vi "novatel_bestvel.vi"(11 "gps_data":u8[](array[numeric])=[170, 68, 18, 28, 42, 0, 2, 32, 72, 0, 0, 0, 144, 180, 147, 5, 176, 171, 185, 18, 0, 0, 0, 0, 69, 97, 188, 10, 0, 0, 0, 0, 16, 0, 0, 0, 27, 4, 80, 179, 242, 142, 73, 64, 22, 250, 107, 190, 124, 130, 92, 192, 0, 96, 118, 159, 68, 159, 144, 64, 166, 42, 130, 193, 61, 0, 0, 0, 18, 90, 203, 63, 205, 158, 152, 63, 219, 102, 64, 64, 0, 48, 48, 48, 0, 0, 0, 0, 0, 0, 0, 0, 11, 11, 0, 0, 0, 6, 0, 3, 66, 220, 76, 72]) -> (3 "vel":dbl[](array[numeric]) format="%#_19f")   [LabVIEW 2015]
panel:
  out "checksum":bool
  out "bestvel":T1 {"sol stat" format="%x"; "vel type" format="%x"}
  out "log Header":T2 {"Sync_AA" format="%02x"; "Sync_44" format="%02x"; "Sync_12" format="%02x"; "Message ID" format="%.6f"; "ms" format="%.19f"}
  out "error out":errorcluster
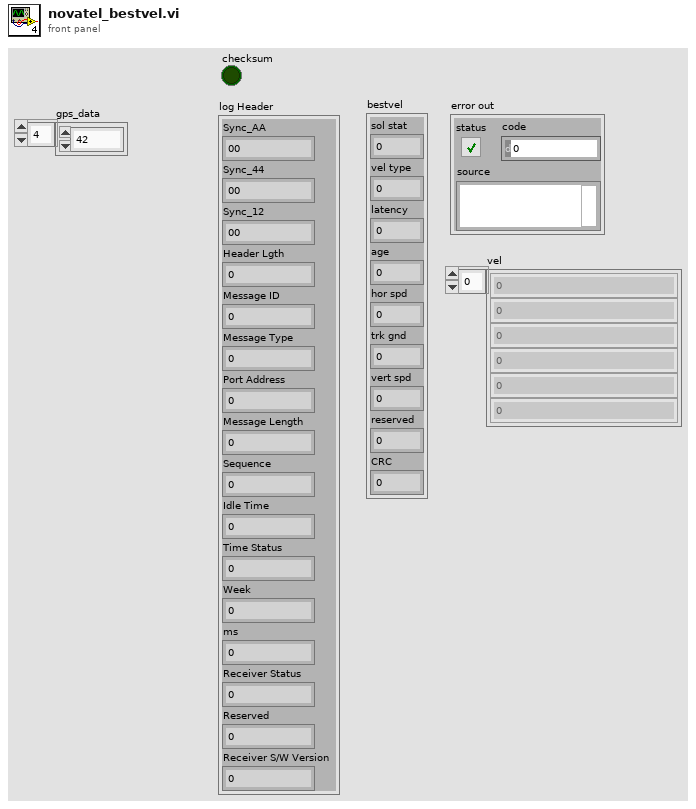
[diagram p1: front panel]
types:
  T1 = cluster{"sol stat":u32, "vel type":u32, "latency":sgl, "age":sgl, "hor spd":dbl, "trk gnd":dbl, "vert spd":dbl, "reserved":sgl, "CRC":u32}
  T2 = cluster{"Sync_AA":u8, "Sync_44":u8, "Sync_12":u8, "Header Lgth":u8, "Message ID":u16, "Message Type":u8, "Port Address":u8, "Message Length":u16, "Sequence":u16, "Idle Time":u8, "Time Status":u8, "Week":u16, "ms":u32, "Receiver Status":u32, "Reserved":u16, "Receiver S/W Version":u16}
  T3 = enum16{"big-endian, network order", "native, host order", "little-endian"}
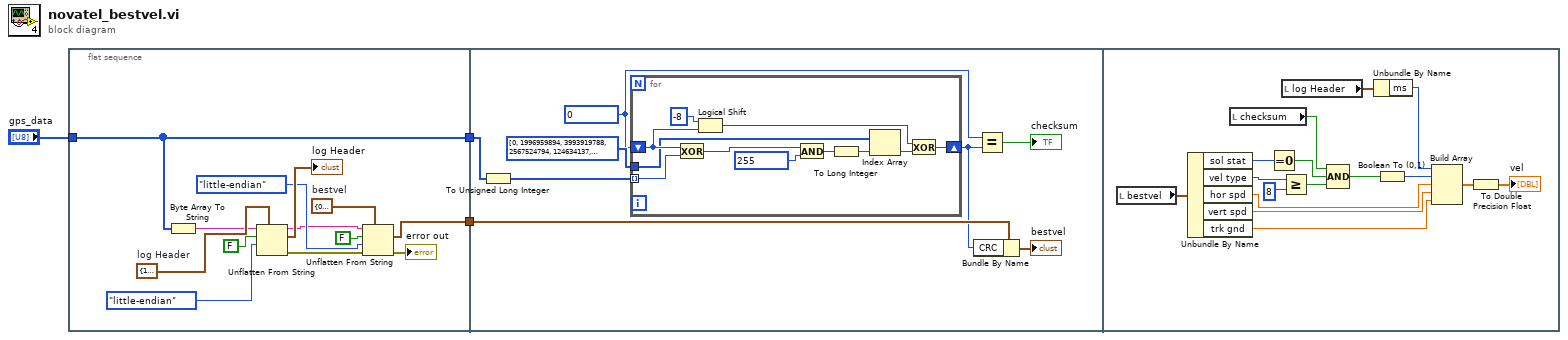
[diagram p0: block diagram]
diagram:
  n1 = flat-sequence {
    tunnel: "gps_data" -> [w7]
    tunnel: [w7] -> w3
    tunnel: [w6] -> w2
    tunnel: w3 -> [w18]
    tunnel: w2 -> [w20]
    frame #0 {
      w4 = T1 {"sol stat"=0, "vel type"=0, "latency"=0.0, "age"=0.0, "hor spd"=0.0, "trk gnd"=0.0, "vert spd"=0.0, "reserved"=0.0, "CRC"=0}  # bestvel
      w16 = T2 {"Sync_AA"=170, "Sync_44"=68, "Sync_12"=18, "Header Lgth"=0, "Message ID"=0, "Message Type"=0, "Port Address"=0, "Message Length"=0, "Sequence"=0, "Idle Time"=0, "Time Status"=0, "Week"=0, "ms"=0, "Receiver Status"=0, "Reserved"=0, "Receiver S/W Version"=0}  # log Header
      n2 = Byte Array To String(unsigned byte array=w7) -> (string=w13:string)
      n3 = Unflatten From String(type=w16, binary string=w13, data includes array or string size? (T)=FALSE, byte order (0:big-endian, network order)=T3."little-endian") -> (rest of the binary string=w10:string, value=→"log Header":T2, error out=w8:errorcluster)  [unwired: 1 in]
      n4 = Unflatten From String(type=w4, binary string=w10, data includes array or string size? (T)=FALSE, byte order (0:big-endian, network order)=T3."little-endian", error in (no error)=w8) -> (value=w6:T1, error out=→"error out":errorcluster)  [unwired: 1 out]
    }
    frame #1 {
      w22 = u32 0
      n5 = To Unsigned Long Integer(number=w18) -> (unsigned 32bit integer=w24:u32[])
      n6 = for {
        shift-right: [w31] -> w19
        shift-left: w22 -> [w34]
        tunnel: w24 -> [w29] mode=indexing
        tunnel: u32[] [0, 1996959894, 3993919788, 2567524794, 124634137, 1886057615, 3915621685, 2657392035, 249268274, 2044508324, 3772115230, 2547177864, 162941995, 2125561021, 3887607047, 2428444049, 498536548, 1789927666, 4089016648, 2227061214, 450548861, 1843258603, 4107580753, 2211677639, 325883990, 1684777152, 4251122042, 2321926636, 335633487, 1661365465, 4195302755, 2366115317, 997073096, 1281953886, 3579855332, 2724688242, 1006888145, 1258607687, 3524101629, 2768942443, 901097722, 1119000684, 3686517206, 2898065728, 853044451, 1172266101, 3705015759, 2882616665, 651767980, 1373503546, 3369554304, 3218104598, 565507253, 1454621731, 3485111705, 3099436303, 671266974, 1594198024, 3322730930, 2970347812, 795835527, 1483230225, 3244367275, 3060149565, 1994146192, 31158534, 2563907772, 4023717930, 1907459465, 112637215, 2680153253, 3904427059, 2013776290, 251722036, 2517215374, 3775830040, 2137656763, 141376813, 2439277719, 3865271297, 1802195444, 476864866, 2238001368, 4066508878, 1812370925, 453092731, 2181625025, 4111451223, 1706088902, 314042704, 2344532202, 4240017532, 1658658271, 366619977, 2362670323, 4224994405, 1303535960, 984961486, 2747007092, 3569037538, 1256170817, 1037604311, 2765210733, 3554079995, 1131014506, 879679996, 2909243462, 3663771856, 1141124467, 855842277, 2852801631, 3708648649, 1342533948, 654459306, 3188396048, 3373015174, 1466479909, 544179635, 3110523913, 3462522015, 1591671054, 702138776, 2966460450, 3352799412, 1504918807, 783551873, 3082640443, 3233442989, 3988292384, 2596254646, 62317068, 1957810842, 3939845945, 2647816111, 81470997, 1943803523, 3814918930, 2489596804, 225274430, 2053790376, 3826175755, 2466906013, 167816743, 2097651377, 4027552580, 2265490386, 503444072, 1762050814, 4150417245, 2154129355, 426522225, 1852507879, 4275313526, 2312317920, 282753626, 1742555852, 4189708143, 2394877945, 397917763, 1622183637, 3604390888, 2714866558, 953729732, 1340076626, 3518719985, 2797360999, 1068828381, 1219638859, 3624741850, 2936675148, 906185462, 1090812512, 3747672003, 2825379669, 829329135, 1181335161, 3412177804, 3160834842, 628085408, 1382605366, 3423369109, 3138078467, 570562233, 1426400815, 3317316542, 2998733608, 733239954, 1555261956, 3268935591, 3050360625, 752459403, 1541320221, 2607071920, 3965973030, 1969922972, 40735498, 2617837225, 3943577151, 1913087877, 83908371, 2512341634, 3803740692, 2075208622, 213261112, 2463272603, 3855990285, 2094854071, 198958881, 2262029012, 4057260610, 1759359992, 534414190, 2176718541, 4139329115, 1873836001, 414664567, 2282248934, 4279200368, 1711684554, 285281116, 2405801727, 4167216745, 1634467795, 376229701, 2685067896, 3608007406, 1308918612, 956543938, 2808555105, 3495958263, 1231636301, 1047427035, 2932959818, 3654703836, 1088359270, 936918000, 2847714899, 3736837829, 1202900863, 817233897, 3183342108, 3401237130, 1404277552, 615818150, 3134207493, 3453421203, 1423857449, 601450431, 3009837614, 3294710456, 1567103746, 711928724, 3020668471, 3272380065, 1510334235, 755167117] ("Array") -> [w25]
        n7 = Exclusive Or(1:w29, 2:w34) -> (0:w33:u32)
        n8 = Logical Shift(y=i16 -8, x=w34) -> (x << y=w30:u32)
        n9 = And(x=w33, y=u32 255) -> (x .and. y?=w28:u32)
        n10 = To Long Integer(number=w28) -> (32bit integer=w27:i32)
        n11 = Index Array(array=w25, index=w27) -> (element=w26:u32)
        n12 = Exclusive Or(1:w26, 2:w30) -> (0:w31:u32)
      }
      n13 = Bundle By Name(cluster=w20, "CRC"=w19) -> (→"bestvel":T1)
      n14 = Equal?(x=w22, y=w19) -> (x = y?=→"checksum":bool)
    }
    frame #2 {
      n15 = local read "bestvel"() -> (w43:T1)
      n16 = Unbundle By Name(w43) -> ("sol stat"=w42:u32, "vel type"=w41:u32, "hor spd"=w51:dbl, "vert spd"=w50:dbl, "trk gnd"=w49:dbl)
      n17 = local read "checksum"() -> (w40:bool)
      n18 = Equal To 0?(x=w42) -> (x = 0?=w39:bool)
      n19 = Greater Or Equal?(x=w41, y=u32 8) -> (x >= y?=w38:bool)
      n20 = local read "log Header"() -> (w47:T2)
      n21 = Compound Arithmetic op=AND(w40, w39, w38) -> (w37:bool)
      n22 = Unbundle By Name(w47) -> ("ms"=w46:u32)
      n23 = Boolean To (0,1)(Boolean=w37) -> (0, 1=w36:i16)
      n24 = Build Array(w46, w36, w51, w50, w49) -> (w48:dbl[])
      n25 = To Double Precision Float(number=w48) -> (double precision float=→"vel":dbl[])
    }
  }
